vi "Main.vi"(11 "Module Admin":refnum<class "Delacor_lib_QMH_Module Admin.lvclass">) -> ()   [LabVIEW 2024, in "Acquisition.lvlib"]
doc: "This template is based off of the Queued Message Handler design pattern and the Queued Message Handler project template that ships with LabVIEW.\n\nThe main difference is that the queue is private to this module and communication between modules is performed via Broadcast and Request events.\n\nRequest events are wrapped in public API methods and are handled in the Event Handling Loop (EHL) of this VI. Any module can register for Broadcast events sent by this module. The EHL generates messages based on user interface actions.\n\nThe Message Handling Loop (MHL) processes messages generated by the EHL, or by other messages. The messages are string values, so new messages can be added easily to the Message Cases case structure in the MHL. Each message cluster can also provide an optional value for Message Data, which is a variant that can be converted to whatever message-specific data is required.\n_____\nBased on DQMH Project Template 4.0.0.47.\n_____\nBased on DQMH Dev Tools: Project Template 7.1.0.1503."
uses:
  Acquisition.lvlib
  <vilib>/Delacor/Delacor QMH/Libraries/Module Admin_class/Delacor_lib_QMH_Module Admin.lvclass
  Module Data--cluster.ctl
  CML Shared/Signal Type--enum.ctl
  CML Shared/Calibration Values--cluster.ctl
  Stop Argument--cluster.ctl
  <vilib>/Delacor/Delacor QMH/Libraries/Message Queue_class/Delacor_lib_QMH_Message Queue.lvclass/Delacor_lib_QMH_Message Queue.ctl
  <vilib>/Delacor/Delacor QMH/Libraries/Module Admin_class/Delacor_lib_QMH_Module Admin.lvclass/Delacor_lib_QMH_Module Admin.ctl
  Start Acquiring Argument--cluster.ctl
  Start Acquiring (Reply Payload)--cluster.ctl
  Stop Acquiring Argument--cluster.ctl
  Settings Editor/Update Application Settings (Reply Payload)--cluster.ctl
  Settings Editor/Settings--cluster.ctl
  <vilib>/Utility/miscctls.llb/LVPointTypeDef.ctl
  <vilib>/Delacor/Delacor QMH/Libraries/Message Queue_class/Delacor_lib_QMH_Enqueue Message (Single).vi
  <vilib>/Delacor/Delacor QMH/Libraries/Module Admin_class/Delacor_lib_QMH_Get External Launch.vi
  <vilib>/Delacor/Delacor QMH/Libraries/Message Queue_class/Delacor_lib_QMH_Message Queue.lvclass
  CML Shared/CML Shared.lvlib
  Settings Editor/Settings Editor.lvlib
  Logger/Logger.lvlib
panel:
  out "Settings":T1
  out "Graph Data":waveform(dbl)[](array[waveform])
  out "error out":errorcluster
  # "This is a headless module. Show its panel to confirm that the Settings are updated correctly and other debugging tasks. Use the Settings Editor to change the settings for this module."
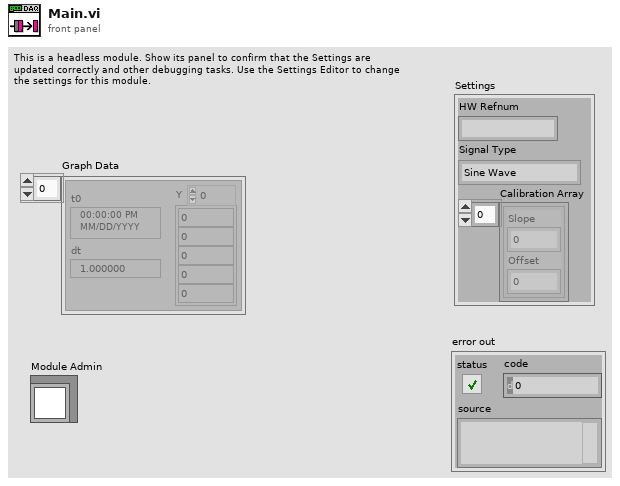
[diagram p1: front panel]
types:
  T1 = typedef "Acquisition.lvlib/Module Data--cluster.ctl" = cluster{"HW Refnum":string, "Signal Type":T2, "Calibration Array":T3[]}
  T2 = typedef "CML Shared.lvlib/Signal Type--enum.ctl" = enum16{"Sine Wave", "Square with Noise"}
  T3 = typedef "CML Shared.lvlib/Calibration Values--cluster.ctl" = cluster{"Slope":dbl, "Offset":dbl}
  T4 = typedef "Settings Editor.lvlib/Broadcast Events--cluster.ctl" = cluster{"Module Did Init":refnum<user-event>, "Status Updated":refnum<user-event>, "Error Reported":refnum<user-event>, "Module Did Stop":refnum<user-event>, "Update Module Execution Status":refnum<user-event>, "Application Settings Updated":refnum<user-event>}
  T5 = typedef "Acquisition.lvlib/Request Events--cluster.ctl" = cluster{"Stop Module":refnum<user-event>, "Show Panel":refnum<user-event>, "Hide Panel":refnum<user-event>, "Get Module Execution Status":refnum<user-event>, "Show Diagram":refnum<user-event>, "Stop Acquiring":refnum<user-event>, "Wakeup Helper Loop":refnum<user-event>, "Change Settings":refnum<user-event>, "Calibrate DAQ":refnum<user-event>, "Start Acquiring":refnum<user-event>}
  T6 = enum32{"invalid lock state", "Not Locked", "Locked (No Password)", "Password-protected"}
  T7 = typedef "Acquisition.lvlib/Stop Argument--cluster.ctl" = cluster{"Origin":string, "Exit via Stop Module Req?":bool, "Wait for Module to stop?":bool}
  T8 = typedef "Acquisition.lvlib/Start Acquiring Argument--cluster.ctl" = cluster{"Wait Notifier":refnum<notifier>, "wait for reply":bool}
  T9 = typedef "Acquisition.lvlib/Stop Acquiring Argument--cluster.ctl" = cluster{"Boolean":bool}
  T10 = typedef "Settings Editor.lvlib/Update Application Settings (Reply Payload)--cluster.ctl" = cluster{"Settings":T11, "error":errorcluster}
  T11 = typedef "Settings Editor.lvlib/Settings--cluster.ctl" = cluster{"Signal Type":T2, "Calibration Array":T3[], "Log File Base Path":path}
  T12 = typedef "LVPointTypeDef.ctl" = cluster{"Horizontal":i16, "Vertical":i16}
  T13 = enum32{"Invalid", "Standard", "Closed", "Hidden", "Minimized", "Maximized"}
  T14 = typedef "Acquisition.lvlib/Start Acquiring (Reply Payload)--cluster.ctl" = cluster{"HW ID":string, "error":errorcluster}
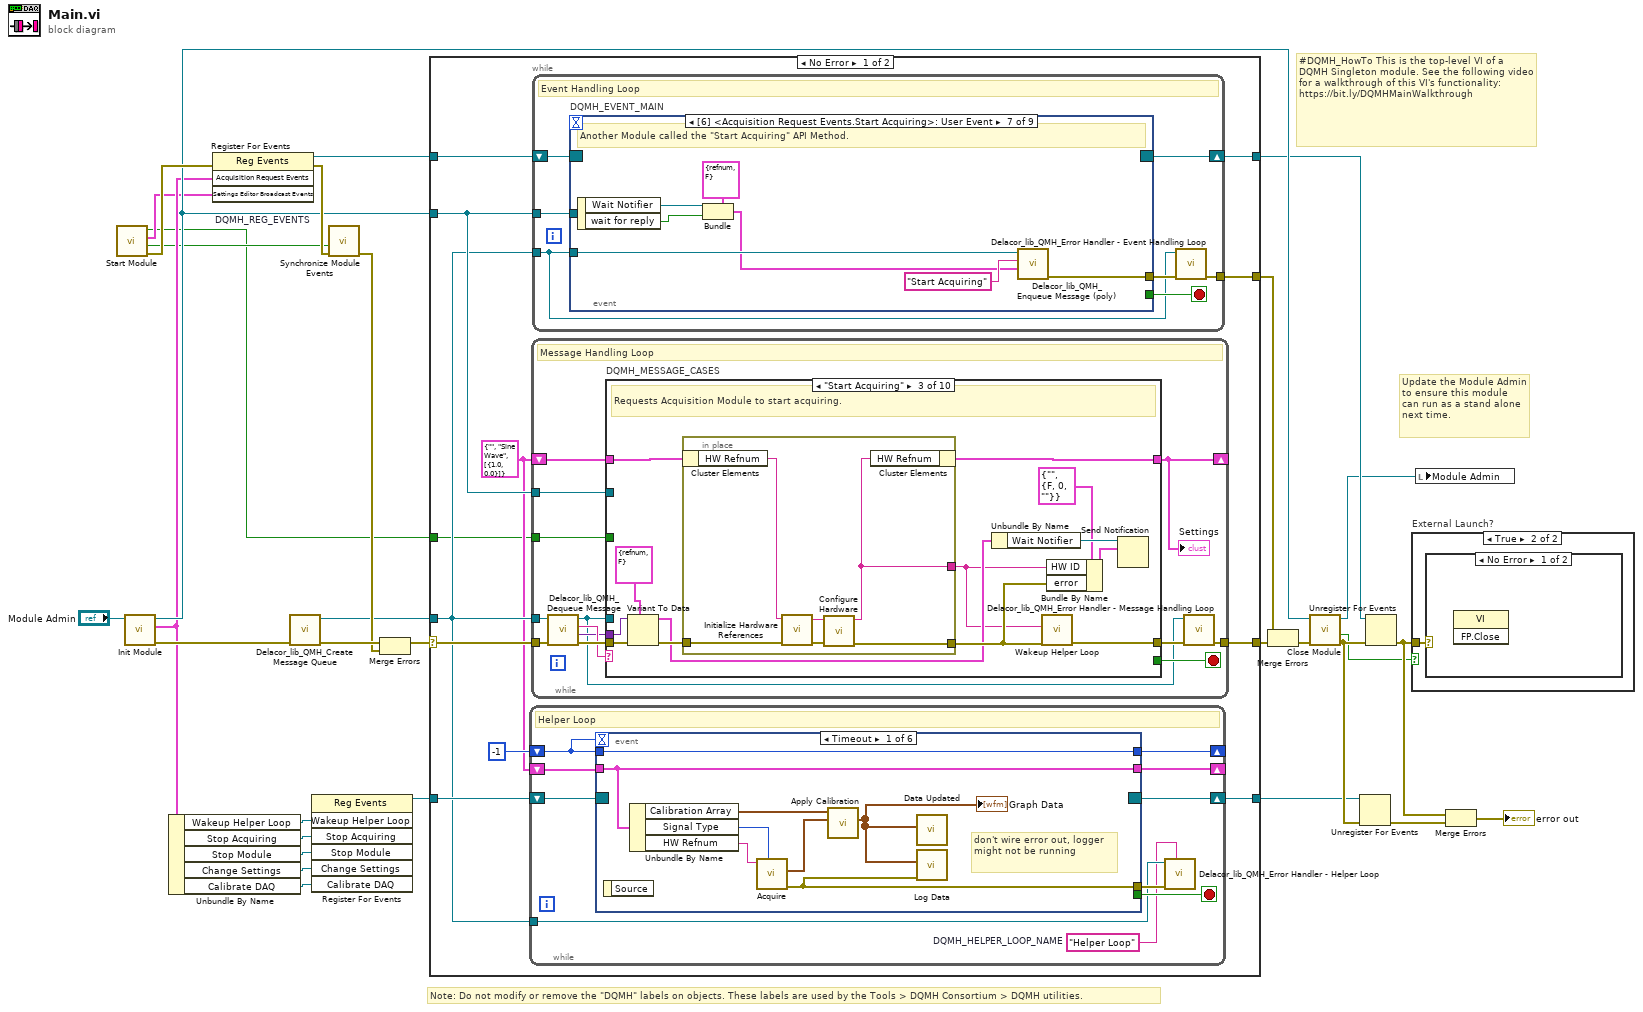
[diagram p0: block diagram]
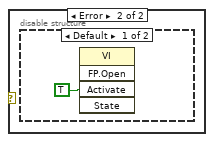
[diagram p3: hidden frame]
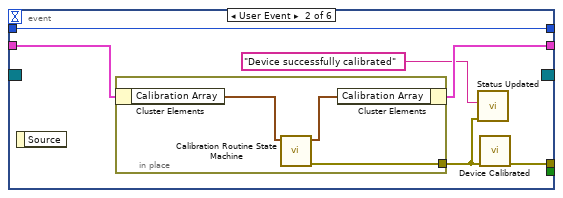
[diagram p5: hidden frame]
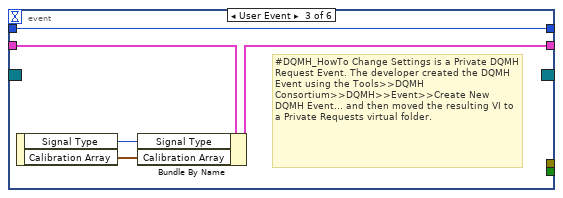
[diagram p6: hidden frame]
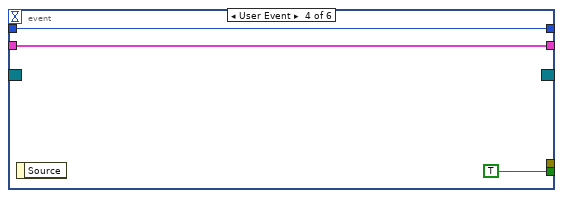
[diagram p7: hidden frame]
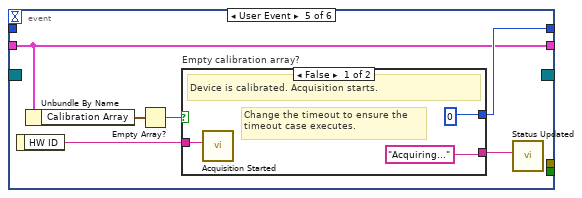
[diagram p8: hidden frame]
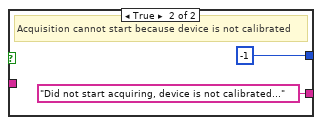
[diagram p9: hidden frame]
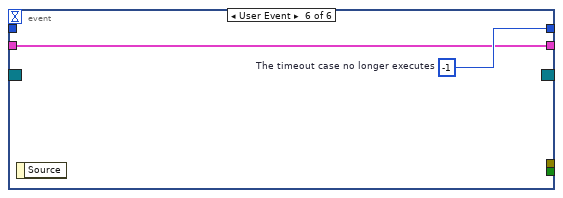
[diagram p10: hidden frame]
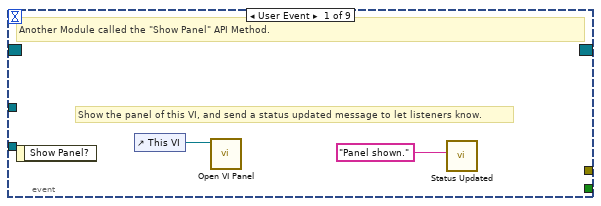
[diagram p11: hidden frame]
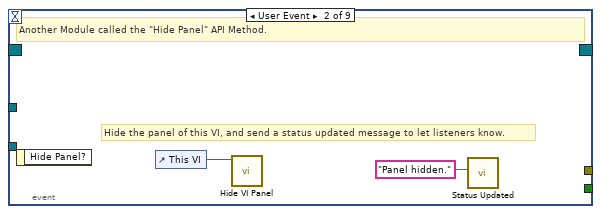
[diagram p12: hidden frame]
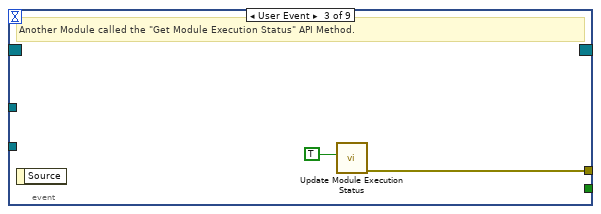
[diagram p13: hidden frame]
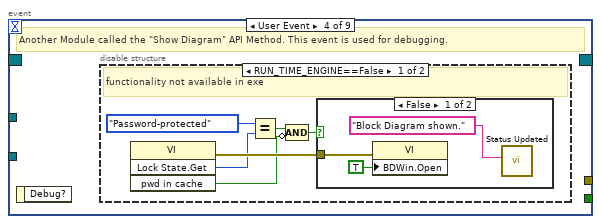
[diagram p14: hidden frame]
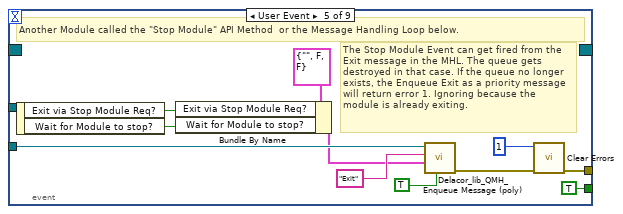
[diagram p17: hidden frame]
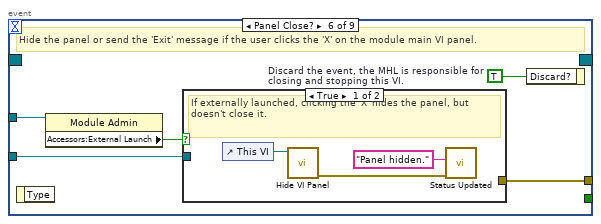
[diagram p18: hidden frame]
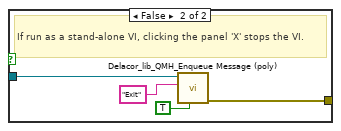
[diagram p19: hidden frame]
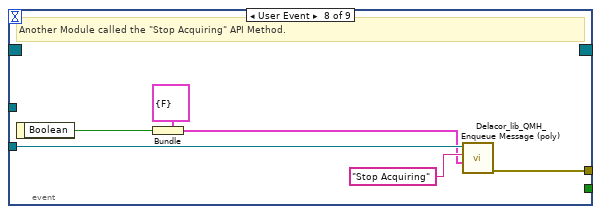
[diagram p20: hidden frame]
diagram:
  # "#DQMH_HowTo This is the top-level VI of a DQMH Singleton module. See the following video for a walkthrough of this VI's functionality: https://bit.ly/DQMHMainWalkthrough"
  # "Note: Do not modify or remove the \"DQMH\" labels on objects. These labels are used by the Tools > DQMH Consortium > DQMH utilities."
  # "Update the Module Admin to ensure this module can run as a stand alone next time."
  n1 = call "Start Module.vi"() -> ("error out"=w24:errorcluster, "Wait for Event Sync?"=w5:bool, "Settings Editor Broadcast Events"=w6:T4, "Module Was Already Running?"=w1:bool)  [unwired: 7 in, 1 out]
  n2 = call "Init Module.vi"("Singleton Module Admin in"="Module Admin") -> ("error out"=w30:errorcluster, "Acquisition Request Events"=w11:T5, "Singleton Module Admin out"=w18:refnum<class "Delacor_lib_QMH_Module Admin.lvclass">)  [unwired: 8 in]
  n3 = Unbundle By Name(w11) -> ("Wakeup Helper Loop"=w7:refnum<user-event>, "Stop Acquiring"=w10:refnum<user-event>, "Stop Module"=w9:refnum<user-event>, "Change Settings"=w4:refnum<user-event>, "Calibrate DAQ"=w3:refnum<user-event>)
  n4 = register-events "DQMH_REG_EVENTS"(error in=w24, w11, w6) -> (reference out=w16:refnum<event-registration>, error out=w23:errorcluster)  [unwired: 1 in]
  n5 = call <vilib>:"Delacor_lib_QMH_Create Message Queue.vi"("error in"=w30) -> ("error out"=w26:errorcluster, "Message Queue"=w15:refnum<class "Delacor_lib_QMH_Message Queue.lvclass">)  [unwired: 9 in]
  n6 = register-events(w7, w10, w9, w4, w3) -> (reference out=w8:refnum<event-registration>)  [unwired: 2 in, 1 out]
  n7 = call "Synchronize Module Events.vi"("error in"=w23, "Wait for Event Sync?"=w5) -> ("error out"=w22:errorcluster)  [unwired: 9 in]
  n8 = Merge Errors(w26, w22) -> (w25:errorcluster)
  n9 = case shown="No Error" w25 {
    selector: w25 -> [w41 w294]
    tunnel: [w43 w293] -> w31
    tunnel: [w40 w292] -> w17
    tunnel: w16 -> [w39 w292]
    tunnel: w15 -> [w35 w285]
    tunnel: [w42 _] -> w29
    tunnel: w18 -> [w38 w288]
    tunnel: w8 -> [w36 w287]
    tunnel: [w33 w287] -> w2
    tunnel: w1 -> [w32 w286]
    frame No Error {
      w34 = T1 {"HW Refnum"="", "Signal Type"=enum."Sine Wave", "Calibration Array"=[{"Slope"=1.0, "Offset"=0.0}]} ("Data Cluster")
      n10 = while {
        shift-right: [w52] -> _
        shift-left: -1 -> [w51]
        tunnel: w35 -> [w45]
        shift-right: [w48] -> _
        shift-left: w34 -> [w47]
        shift-right: [w46] -> w33
        shift-left: w36 -> [w50]
        stop <- w49 stop-if-true
        w44 = "Helper Loop"  # DQMH_HELPER_LOOP_NAME
        # "Helper Loop"
        n11 = event shown="[0] Timeout" {
          selector: w50 -> [_ _ _ _ _ _]
          dyn-events: [_ _ _ _ _ _] -> w46
          timeout: w51 -> [_ _ _ _ _ _]
          tunnel: [w60 w65 w75 w78 w83 w91] -> w52
          tunnel: w51 -> [w60 w65 w75 w78 _ _]
          tunnel: [_ _ _ TRUE _ _] -> w49
          tunnel: [w61 w67 _ _ _ _] -> w53
          tunnel: [w57 w63 w73 w76 w80 w90] -> w48
          tunnel: w47 -> [w57 w64 w74 w76 w80 w90]
          event Timeout {
            # "don't wire error out, logger might not be running"
            n12 = event-data() -> ()  [unwired: 1 in, 1 out]
            n13 = Unbundle By Name(w57) -> ("Calibration Array"=w55:T3[], "Signal Type"=w59:T2, "HW Refnum"=w58:string)
            n14 = call "Acquire.vi"("Signal Type"=w59, "HW ID in"=w58) -> ("error out"=w61:errorcluster, "Graph Data"=w56:waveform(dbl)[])  [unwired: 7 in, 1 out]
            n15 = call "Apply Calibration.vi"("Graph Data"=w56, "Calibration Array"=w55) -> ("Calibrated Data"=w54:waveform(dbl)[])  [unwired: 9 in]
            "Graph Data" <- w54
            n16 = call "Data Updated.vi"("Graph Data"=w54) -> ()  [unwired: 10 in, 1 out]
            n17 = call "Log Data.vi"("error in"=w61, "Waveforms"=w54) -> ()  [unwired: 9 in, 1 out]
          }
          event User Event {
            n18 = event-data() -> ()  [unwired: 1 in, 1 out]
            n19 = in-place {
              in-place-border: [w70] -> w66
              n20 = in-place-cluster #1(w64) -> ("Calibration Array"=w69:T3[])
              n21 = call "Calibration Routine State Machine.vi"("Calibration Array in"=w69) -> ("error out"=w70:errorcluster, "Calibration Array out"=w68:T3[])  [unwired: 9 in]
              n22 = in-place-cluster #1("Calibration Array"=w68) -> (w63:T1)
            }
            n23 = call "Status Updated.vi"("error in"=w66, "Status"="Device successfully calibrated") -> ()  [unwired: 9 in, 1 out]
            n24 = call "Device Calibrated.vi"("error in"=w66) -> ("error out"=w67:errorcluster)  [unwired: 10 in]
          }
          event User Event {
            # "#DQMH_HowTo Change Settings is a Private DQMH Request Event. The developer created the DQMH Event using the Tools>>DQMH Consortium>>DQMH>>Event>>Create New DQMH Event... and then moved the resulting VI to a Private Requests virtual folder."
            n25 = event-data() -> ("Signal Type"=w72:T2, "Calibration Array"=w71:T3[])  [unwired: 1 in]
            n26 = Bundle By Name(cluster=w74, "Signal Type"=w72, "Calibration Array"=w71) -> (w73:T1)
          }
          event User Event {
            n27 = event-data() -> ()  [unwired: 1 in, 1 out]
          }
          event User Event {
            n28 = event-data() -> ("HW ID"=w81:string)  [unwired: 1 in]
            n29 = Unbundle By Name(w80) -> ("Calibration Array"=w79:T3[])
            n30 = Empty Array?(array=w79) -> (empty?=w84:bool)
            n31 = case "Empty calibration array?" shown="False" w84 {
              tunnel: ["Acquiring..." ("Status") "Did not start acquiring, device is not calibrated..." ("Status")] -> w82
              tunnel: [0 -1] -> w83
              tunnel: w81 -> [w87 _]
              frame False {
                # "Change the timeout to ensure the timeout case executes."
                # "Device is calibrated. Acquisition starts."
                n32 = call "Acquisition Started.vi"("HW ID"=w87) -> ()  [unwired: 10 in, 1 out]
              }
              frame True {
                # "Acquisition cannot start because device is not calibrated"
              }
            }
            n33 = call "Status Updated.vi"("Status"=w82) -> ()  [unwired: 10 in, 1 out]
          }
          event User Event {
            w91 = -1  # The timeout case no longer executes
            n34 = event-data() -> ()  [unwired: 1 in, 1 out]
          }
        }
        n35 = call-dynamic "Delacor_lib_QMH_Error Handler - Helper Loop.vi"("Error Debug"=w44, "error in"=w53, "Message Queue in"=w45) -> ()  [unwired: 7 in, 2 out]
      }
      n36 = while {
        tunnel: w35 -> [w159]
        shift-right: [w163] -> _
        shift-left: w34 -> [w164]
        tunnel: w41 -> [w167]
        tunnel: [w165] -> w43
        tunnel: w38 -> [w157]
        tunnel: w32 -> [w156]
        stop <- w162 stop-if-true
        # "Message Handling Loop"
        n37 = call-dynamic "Delacor_lib_QMH_Dequeue Message.vi"("error in"=w167, "Message Queue in"=w159) -> ("error out"=w166:errorcluster, "Message Data"=w160:variant, "Message"=w161:string, "Message Queue out"=w158:refnum<class "Delacor_lib_QMH_Message Queue.lvclass">)  [unwired: 6 in]
        n38 = case "DQMH_MESSAGE_CASES" shown="\"Start Acquiring\"" w161 {
          selector: w161 -> [_ _ _ _ _ _ _ _ _ w280]
          tunnel: w158 -> [_ _ _ _ _ _ _ w241 w265 _]
          tunnel: w166 -> [w191 w195 w208 w222 w232 w235 w237 w248 w272 w283]
          tunnel: [w172 w195 w206 w220 w230 w234 w237 w244 w266 w284] -> w168
          tunnel: w164 -> [w182 w194 w196 w217 w228 w233 w236 w243 w257 w281]
          tunnel: [w177 w194 w204 w217 w228 w233 w236 w243 w257 w281] -> w163
          tunnel: [_ _ _ _ _ _ _ _ w264 _] -> w162
          tunnel: w160 -> [_ _ w203 w219 w229 _ _ w242 w263 _]
          tunnel: w157 -> [w183 _ _ _ _ _ _ w240 w258 _]
          tunnel: w156 -> [_ _ _ _ _ _ _ _ w255 _]
          frame "Initialize" {
            # "Initialize - Any operation that needs to be done before the module can receive messages. Synchronize Caller Events.vi will inform Start Module.vi that the module has launched and is ready to receive messages. Module Did Init.vi will broadcast that the module initialized."
            n39 = call "Synchronize Caller Events.vi"("error in"=w191, "Singleton Module Admin in"=w183) -> ("error out"=w170:errorcluster, "Singleton Module Admin out"=w179:refnum<class "Delacor_lib_QMH_Module Admin.lvclass">)  [unwired: 8 in]
            n40 = call "Update Application Settings.vi"("wait for reply (T)"=TRUE) -> ("error out"=w169:errorcluster, "Reply Payload"=w176:T10)  [unwired: 8 in, 1 out]
            n41 = property on="Property Node" class="Module Admin"(reference=w179) -> ("Accessors:External Launch"=w187:bool)  [unwired: 1 in, 2 out]
            n42 = Unbundle By Name(w176) -> ("Settings.Signal Type"=w175:T2, "Settings.Calibration Array"=w174:T3[])
            n43 = Select(t=T13."Hidden" ("State"), s=w187, f=T13."Standard" ("State")) -> (s? t:f=w184:T13)
            n44 = Merge Errors(w170, w169) -> (w171:errorcluster)
            n45 = Bundle By Name(cluster=w182, "Signal Type"=w175, "Calibration Array"=w174) -> (w177:T1)
            n46 = call "Module Name--constant.vi"() -> ("Module Name"=w190:string)  [unwired: 11 in]
            n47 = property on="Property Node" class="VI"("Front Panel.Title"=w190) -> (reference out=w189:refnum<vi>, error out=w193:errorcluster)  [unwired: 2 in]
            n48 = invoke on="Invoke Node" class="VI" method="FP.Open"(reference=w189, error in=w193, "State"=w184) -> (reference out=w188:refnum<vi>, error out=w192:errorcluster)  [unwired: 2 in, 3 out]
            n49 = call "Module Name--constant.vi"() -> ("Module Name"=w180:string)  [unwired: 11 in]
            n50 = invoke on="Invoke Node" class="VI" method="FP.Center"(reference=w188, error in=w192) -> ()  [unwired: 1 in, 3 out]
            n51 = property on="Pane" class="Pane"("Origin"=T12 {"Horizontal"=0, "Vertical"=0}) -> ()  [unwired: 2 in, 2 out]
            n52 = call "Module Did Init.vi"("error in"=w171, "Initialized?"=TRUE, "Origin"=w180) -> ("error out"=w172:errorcluster)  [unwired: 8 in]
          }
          frame "---Module Specific---" {
            # "Separator -- The following cases handle messages specific to this Module."
          }
          frame "Start Acquiring" {
            # "Requests Acquisition Module to start acquiring."
            n53 = Variant To Data(error in=w208, type=T8 {"Wait Notifier"=refnum, "wait for reply"=FALSE} ("Start Acquisition Argument"), Variant=w203) -> (data=w201:T8, error out=w205:errorcluster)
            n54 = in-place {
              in-place-border: [w214] -> w207
              in-place-border: w205 -> [w213]
              in-place-border: [w209] -> w197
              n55 = in-place-cluster #2(w196) -> ("HW Refnum"=w210:string)
              n56 = call "Initialize Hardware References.vi"("error in"=w213, "HW Refnum in"=w210) -> ("error out"=w212:errorcluster, "HW Refnum out"=w211:string)  [unwired: 8 in]
              n57 = call "Configure Hardware.vi"("error in"=w212, "HW Refnum in"=w211) -> ("error out"=w214:errorcluster, "HW Refnum out"=w209:string)  [unwired: 8 in]
              n58 = in-place-cluster #2("HW Refnum"=w209) -> (w204:T1)
            }
            n59 = Unbundle By Name(w201) -> ("Wait Notifier"=w200:refnum<notifier>)
            n60 = call "Wakeup Helper Loop.vi"("error in"=w207, "HW ID"=w197) -> ("error out"=w206:errorcluster)  [unwired: 9 in]
            n61 = Bundle By Name(cluster=T14 {"HW ID"="", "error"={"status"=FALSE, "code"=0, "source"=""}} ("Start Acquisition (Reply Payload)"), "HW ID"=w197, "error"=w207) -> (w199:T14)
            n62 = Send Notification(notification=w199, notifier=w200) -> ()  [unwired: 1 in, 2 out]
          }
          frame "Stop Acquiring" {
            # "Requests the Acquisition Module to stop acquiring"
            n63 = Variant To Data(error in=w222, type=T9 {"Boolean"=FALSE} ("Stop Acquiring Argument"), Variant=w219) -> (error out=w221:errorcluster)  [unwired: 1 out]
            n64 = Unbundle By Name(w217) -> ("HW Refnum"=w216:string)
            n65 = call "Stop Acquisition.vi"("error in"=w221, "HW Refnum"=w216) -> ("error out"=w220:errorcluster)  [unwired: 9 in]
            n66 = call "Acquisition Stopped.vi"("error in"=w220) -> ()  [unwired: 10 in, 1 out]
            n67 = call "Status Updated.vi"("error in"=w220, "Status"="Acquisition Stopped") -> ()  [unwired: 9 in, 1 out]
          }
          frame "Update Settings" {
            # "Send the Change Settings event to the helper loop."
            # "The Settings Editor broadcasted that the settings have changed."
            n68 = Variant To Data(error in=w232, type=T10 {"Settings"={"Signal Type"=enum."Sine Wave", "Calibration Array"=[], "Log File Base Path"=path ""}, "error"={"status"=FALSE, "code"=0, "source"=""}} ("Settings Updated Argument"), Variant=w229) -> (data=w226:T10, error out=w231:errorcluster)
            n69 = Unbundle By Name(w226) -> ("Settings.Signal Type"=w225:T2, "Settings.Calibration Array"=w223:T3[])
            n70 = call "Change Settings.vi"("error in"=w231, "Calibration Array"=w223, "Signal Type"=w225) -> ("error out"=w230:errorcluster)  [unwired: 8 in]
            n71 = call "Status Updated.vi"("error in"=w230, "Status"="Settings Updated") -> ()  [unwired: 9 in, 1 out]
          }
          frame "---Copy This Frame---" {
            # "Duplicate this frame when creating new messages.  Change this comment in the duplicated frame to describe this message."
            n72 = Merge Errors(w235) -> (w234:errorcluster)
          }
          frame "---Exit and Error Handling---" {
            # "Separator - The following cases handle errors and exit messages."
          }
          frame "Error" {
            # "Error - Check the error message data and respond accordingly. This message is sent by the \"Error Handler\" VIs at the end of each loop in this application."
            n73 = property on="Property Node" class="Module Admin"(reference=w240) -> ("Accessors:External Launch"=w239:bool)  [unwired: 1 in, 2 out]
            n74 = Variant To Data(error in=w248, type=errorcluster {"status"=FALSE, "code"=0, "source"=""} ("error constant"), Variant=w242) -> (data=w238:errorcluster, error out=w246:errorcluster)
            n75 = local write "error out"(w238) -> ()
            n76 = call "Error Reported.vi"("Error"=w238) -> ()  [unwired: 10 in, 1 out]
            n77 = case shown="False" w239 {
              tunnel: [w253 _] -> w245
              tunnel: w241 -> [w251 _]
              tunnel: w238 -> [w252 _]
              frame False {
                n78 = disable-structure shown="Default" {
                  disable-tunnel: w252 -> [w254 _]
                  frame condition #0 (active) {
                    # "If the module is running standalone, then pop up an error dialog and call the \"Exit\" message."
                    n79 = call <vilib>:"Simple Error Handler.vi"("error in (no error)"=w254) -> ()  [unwired: 4 in, 5 out]
                  }
                  frame condition #1 {
                    # "To prevent the Simple Error Handler VI from being loaded (e.g. when deploying to a Real-Time target), add the Conditional Disable Symbol \"DQMH_Disable_SEH\" to your project and set it to TRUE."
                  }
                }
                n80 = call-poly <vilib>:"Delacor_lib_QMH_Enqueue Message (poly).vi"("Priority Message? (F)"=TRUE, "Message"="Exit", "Message Queue in"=w251) -> ("error out"=w253:errorcluster)  [unwired: 7 in, 1 out]
              }
              frame True {
                # "If the module was launched externally, calling the Error Reported broadcast VI is the only action performed by the \"Error\" message. The module's caller can then process the error appropriately."
              }
            }
            n81 = Merge Errors(w246, w245) -> (w244:errorcluster)
          }
          frame "Exit" {
            w264 = TRUE  # Stop the VI
            # "Release the message queue reference"
            # "Exit - Exit the application."
            n82 = Variant To Data(error in=w272, type=T7 {"Origin"="", "Exit via Stop Module Req?"=FALSE, "Wait for Module to stop?"=FALSE} ("Stop Argument"), Variant=w263) -> (data=w260:T7, error out=w269:errorcluster)
            n83 = call <vilib>:"Clear Errors.vi"("error in (no error)"=w269, "specific error code to clear (0: all)"=91 ("91: not all Exit messages will have an argument")) -> ("error out"=w271:errorcluster)  [unwired: 4 in, 1 out]
            n84 = Unbundle By Name(w257) -> ("HW Refnum"=w256:string)
            n85 = control-ref of="This VI"() -> (w259:refnum<vi>)
            n86 = call "Handle Exit.vi"("Stop Argument"=w260, "Admin in"=w258, "VI reference"=w259) -> ("error out"=w268:errorcluster)  [unwired: 7 in, 1 out]
            n87 = call "Close Hardware References.vi"("HW Refnum in"=w256) -> ("error out"=w267:errorcluster)  [unwired: 9 in, 1 out]
            n88 = call-dynamic "Delacor_lib_QMH_Release Message Queue.vi"("error in"=w271, "Message Queue"=w265) -> ("error out"=w270:errorcluster)  [unwired: 9 in]
            n89 = case "Settings Editor was\nalready running?" shown="False" w255 {
              frame False {
                n90 = call "Module Name--constant.vi"() -> ("Module Name"=w274:string)  [unwired: 11 in]
                n91 = call "Stop Module.vi"("Wait for Module to Stop? (F)"=TRUE, "Origin"=w274) -> ()  [unwired: 9 in, 1 out]
              }
              frame True {
                # "Another Module stops the Settings Editor"
              }
            }
            n92 = Merge Errors(w270, w268, w267) -> (w266:errorcluster)
            n93 = call "Error Reported.vi"("Error"=w266) -> ()  [unwired: 10 in, 1 out]
          }
          frame Default {
            # "'Default' case only runs if there is a message that isn't defined in any of the other cases.  Output a programming error."
            n94 = call "Module Name--constant.vi"() -> ("Module Name"=w279:string)  [unwired: 11 in]
            n95 = Format Into String(format string="The invalid message string \"%s\" was received in the Message Handling Loop for module \"%s\".", w280, w279) -> (resulting string=w277:string)  [unwired: 2 in, 1 out]
            n96 = call <vilib>:"Error Cluster From Error Code.vi"("show call chain? (False)"=TRUE, "error message (\"\")"=w277, "error code (0)"=1) -> ("error out"=w282:errorcluster)  [unwired: 6 in]
            n97 = Merge Errors(w283, w282) -> (w284:errorcluster)
          }
        }
        "Settings" <- w163
        n98 = call-dynamic "Delacor_lib_QMH_Error Handler - Message Handling Loop.vi"("error in"=w168, "Message Queue in"=w158) -> ("dup error in"=w165:errorcluster)  [unwired: 8 in, 1 out]
      }
      n99 = while {
        tunnel: w35 -> [w92]
        shift-right: [w95] -> w40
        shift-left: w39 -> [w96]
        tunnel: [w97] -> w42
        tunnel: w38 -> [w93]
        stop <- w94 stop-if-true
        # "Event Handling Loop"
        n100 = event "DQMH_EVENT_MAIN" shown="[6] <Acquisition Request Events.Start Acquiring>: User Event" {
          selector: w96 -> [_ _ _ _ _ _ _ _ _]
          dyn-events: [_ _ _ _ _ _ _ _ _] -> w95
          timeout: _ -> [_ _ _ _ _ _ _ _ _]
          tunnel: [_ _ _ _ TRUE ("Discard?") _ _ _ _] -> w94
          tunnel: w92 -> [_ _ _ _ w120 w127 w142 w148 w153]
          tunnel: [_ _ w104 _ w123 w129 w143 w149 w155] -> w98
          tunnel: w93 -> [_ _ _ _ _ w126 _ _ _]
          event User Event {
            # "Show the panel of this VI, and send a status updated message to let listeners know."
            # "Another Module called the \"Show Panel\" API Method."
            n101 = event-data() -> ()  [unwired: 1 in, 1 out]
            n102 = control-ref of="This VI"() -> (w100:refnum<vi>)
            n103 = call "Open VI Panel.vi"("VI"=w100) -> ()  [unwired: 10 in, 1 out]
            n104 = call "Status Updated.vi"("Status"="Panel shown." ("format string")) -> ()  [unwired: 10 in, 1 out]
          }
          event User Event {
            # "Hide the panel of this VI, and send a status updated message to let listeners know."
            # "Another Module called the \"Hide Panel\" API Method."
            n105 = event-data() -> ()  [unwired: 1 in, 1 out]
            n106 = control-ref of="This VI"() -> (w102:refnum<vi>)
            n107 = call "Hide VI Panel.vi"("VI"=w102) -> ()  [unwired: 10 in, 1 out]
            n108 = call "Status Updated.vi"("Status"="Panel hidden." ("format string")) -> ()  [unwired: 10 in, 1 out]
          }
          event User Event {
            # "Another Module called the \"Get Module Execution Status\" API Method."
            n109 = event-data() -> ()  [unwired: 1 in, 1 out]
            n110 = call "Update Module Execution Status.vi"("Running?"=TRUE) -> ("error out"=w104:errorcluster)  [unwired: 10 in]
          }
          event User Event {
            # "Another Module called the \"Show Diagram\" API Method. This event is used for debugging."
            n111 = event-data() -> ()  [unwired: 1 in, 1 out]
            n112 = disable-structure shown="RUN_TIME_ENGINE==False" {
              frame condition #0 (active) {
                # "functionality not available in exe"
                n113 = invoke on="Invoke Node" class="VI" method="Lock State.Get"() -> (error out=w110:errorcluster, "Get Lock State"=w109:T6, "pwd in cache"=w106:bool)  [unwired: 4 in, 1 out]
                n114 = Equal?(x=T6."Password-protected", y=w109) -> (x = y?=w107:bool)
                n115 = Compound Arithmetic op=AND(w107, invert w106) -> (w105:bool)
                n116 = case shown="False" w105 {
                  tunnel: w110 -> [w113 _]
                  frame False {
                    n117 = property on="Property Node" class="VI"(error in=w113, "BDWin.Open"=TRUE ("Block Diagram Window:Open")) -> ()  [unwired: 1 in, 2 out]
                    n118 = call "Status Updated.vi"("Status"="Block Diagram shown." ("format string")) -> ()  [unwired: 10 in, 1 out]
                  }
                  frame True {
                    # "Password-protected VI, and the password is not in the cache. Do not show the diagram."
                  }
                }
              }
              frame condition #1 {
              }
            }
          }
          event User Event {
            # "The Stop Module Event can get fired from the Exit message in the MHL. The queue gets destroyed in that case. If the queue no longer exists, the Enqueue Exit as a priority message will return error 1. Ignoring because the module is already exiting."
            # "Another Module called the \"Stop Module\" API Method  or the Message Handling Loop below."
            n119 = event-data() -> ("Exit via Stop Module Req?"=w116:bool, "Wait for Module to stop?"=w115:bool)  [unwired: 1 in]
            n120 = Bundle By Name(cluster=T7 {"Origin"="", "Exit via Stop Module Req?"=FALSE, "Wait for Module to stop?"=FALSE} ("Stop Argument"), "Exit via Stop Module Req?"=w116, "Wait for Module to stop?"=w115) -> (w114:T7)
            n121 = call-poly <vilib>:"Delacor_lib_QMH_Enqueue Message (poly).vi"("Priority Message? (F)"=TRUE, "Message Data"=w114, "Message"="Exit", "Message Queue in"=w120) -> ("error out"=w124:errorcluster)  [unwired: 6 in, 1 out]
            n122 = call <vilib>:"Clear Errors.vi"("error in (no error)"=w124, "specific error code to clear (0: all)"=1) -> ("error out"=w123:errorcluster)  [unwired: 4 in, 1 out]
          }
          event Panel Close? {
            w128 = TRUE  # Discard the event, the MHL is responsible for closing and stopping this VI.
            # "Hide the panel or send the 'Exit' message if the user clicks the 'X' on the module main VI panel."
            n123 = event-data() -> ()  [unwired: 1 in, 1 out]
            n124 = property on="Property Node" class="Module Admin"(reference=w126) -> ("Accessors:External Launch"=w125:bool)  [unwired: 1 in, 2 out]
            n125 = case shown="True" w125 {
              tunnel: w127 -> [_ w135]
              tunnel: [_ w136] -> w129
              frame True {
                # "If externally launched, clicking the 'X' hides the panel, but doesn't close it."
                n126 = control-ref of="This VI"() -> (w132:refnum<vi>)
                n127 = call "Hide VI Panel.vi"("VI"=w132) -> ("error out"=w130:errorcluster)  [unwired: 10 in]
                n128 = call "Status Updated.vi"("error in"=w130, "Status"="Panel hidden." ("format string")) -> ()  [unwired: 9 in, 1 out]
              }
              frame False {
                # "If run as a stand-alone VI, clicking the panel 'X' stops the VI."
                n129 = call-poly <vilib>:"Delacor_lib_QMH_Enqueue Message (poly).vi"("Priority Message? (F)"=TRUE, "Message"="Exit", "Message Queue in"=w135) -> ("error out"=w136:errorcluster)  [unwired: 7 in, 1 out]
              }
            }
            n130 = event-data ("Event Filter Node")("Discard?"=w128) -> ()  [unwired: 1 in, 1 out]
          }
          event User Event {
            # "Another Module called the \"Start Acquiring\" API Method."
            n131 = event-data() -> ("Wait Notifier"=w138:refnum<notifier>, "wait for reply"=w137:bool)  [unwired: 1 in]
            n132 = Bundle(cluster=T8 {"Wait Notifier"=refnum, "wait for reply"=FALSE} ("Start Acquisition Argument"), "Wait Notifier"=w138, "wait for reply"=w137) -> (w139:T8)
            n133 = call-poly <vilib>:"Delacor_lib_QMH_Enqueue Message (poly).vi"("Message Data"=w139, "Message"="Start Acquiring", "Message Queue in"=w142) -> ("error out"=w143:errorcluster)  [unwired: 7 in, 1 out]
          }
          event User Event {
            # "Another Module called the \"Stop Acquiring\" API Method."
            n134 = event-data() -> ("Boolean"=w144:bool)  [unwired: 1 in]
            n135 = Bundle(cluster=T9 {"Boolean"=FALSE} ("Stop Acquiring Argument"), "Boolean"=w144) -> (w145:T9)
            n136 = call-poly <vilib>:"Delacor_lib_QMH_Enqueue Message (poly).vi"("Message Data"=w145, "Message"="Stop Acquiring", "Message Queue in"=w148) -> ("error out"=w149:errorcluster)  [unwired: 7 in, 1 out]
          }
          event User Event {
            n137 = event-data() -> ("Settings"=w150:T11)  [unwired: 1 in]
            n138 = Bundle By Name(cluster=T10 {"Settings"={"Signal Type"=enum."Sine Wave", "Calibration Array"=[], "Log File Base Path"=path ""}, "error"={"status"=FALSE, "code"=0, "source"=""}} ("Settings Updated Argument"), "Settings"=w150) -> (w152:T10)
            n139 = call-poly <vilib>:"Delacor_lib_QMH_Enqueue Message (poly).vi"("Message Data"=w152, "Message"="Update Settings", "Message Queue in"=w153) -> ("error out"=w155:errorcluster)  [unwired: 7 in, 1 out]
          }
        }
        n140 = call-dynamic "Delacor_lib_QMH_Error Handler - Event Handling Loop.vi"("error in"=w98, "Message Queue in"=w92) -> ("dup error in"=w97:errorcluster)  [unwired: 8 in, 1 out]
      }
    }
    frame Error {
      # "Synchronize Caller Events.vi will inform Start Module.vi that the module has launched and will let the code calling Start Module.vi register for broadcasts and would permit the caller receive the broadcast that an error occurred at launch time."
      n141 = call "Synchronize Caller Events.vi"("Singleton Module Admin in"=w288) -> ("error out"=w295:errorcluster)  [unwired: 9 in, 1 out]
      n142 = call-dynamic "Delacor_lib_QMH_Release Message Queue.vi"("error in"=w294, "Message Queue"=w285) -> ("error out"=w293:errorcluster)  [unwired: 9 in]
      n143 = call "Module Name--constant.vi"() -> ("Module Name"=w291:string)  [unwired: 11 in]
      n144 = case "Settings Editor was\nalready running?" shown="False" w286 {
        frame False {
          n145 = call "Module Name--constant.vi"() -> ("Module Name"=w298:string)  [unwired: 11 in]
          n146 = call "Stop Module.vi"("Wait for Module to Stop? (F)"=TRUE, "Origin"=w298) -> ()  [unwired: 9 in, 1 out]
        }
        frame True {
          # "Another Module is\nin charge of stopping Settings Editor"
        }
      }
      n147 = Format Into String(format string="An error occurred during initialization. %s is no longer running.", w291) -> (resulting string=w289:string)  [unwired: 2 in, 1 out]
      n148 = Merge Errors(w293, w295) -> (w296:errorcluster)
      n149 = call "Error Reported.vi"("Additional Information"=w289, "Error"=w296) -> ()  [unwired: 9 in, 1 out]
    }
  }
  n150 = Merge Errors(w29, w31) -> (w28:errorcluster)
  n151 = call "Close Module.vi"("error in"=w28, "Module Admin in"=w18) -> ("error out"=w21:errorcluster, "External Launch"=w12:bool, "Module Admin out"=w13:refnum<class "Delacor_lib_QMH_Module Admin.lvclass">)  [unwired: 7 in]
  n152 = Unregister For Events(event registration refnum=w2, error in=w21) -> (error out=w19:errorcluster)
  n153 = Unregister For Events(event registration refnum=w17, error in=w21) -> (error out=w27:errorcluster)
  n154 = case "External Launch?" shown="True" w12 {
    tunnel: w27 -> [_ w299]
    frame False {
    }
    frame True {
      n155 = case shown="No Error" w299 {
        frame No Error {
          n156 = invoke on="Invoke Node" class="VI" method="FP.Close"() -> ()  [unwired: 3 in, 3 out]
        }
        frame Error {
          n157 = disable-structure shown="Default" {
            frame condition #0 (active) {
              n158 = invoke class="VI" method="FP.Open"("Activate"=TRUE ("Activate?")) -> ()  [unwired: 4 in, 5 out]
            }
            frame condition #1 {
              # "Don't show panel on error if running inside a built EXE."
            }
          }
        }
      }
    }
  }
  n159 = local write "Module Admin"(w13) -> ()
  n160 = Merge Errors(w27, w19) -> (→"error out":errorcluster)
